vi "Derivative (DVR).vi"(4 "Type":enum16{"dy/dx vs x", "dx/dy vs y"}(ring), 7 "Data Value Reference in":refnum<data-value>, 8 "error in (no error)":errorcluster, 11 "dX in":refnum<data-value>) -> (0 "error out":errorcluster, 3 "dX out":refnum<data-value>)   [LabVIEW 2016, in "Retrieve and Visualize.lvclass"]
uses:
  Retrieve and Visualize.lvclass
  <userlib>/LevyLab/XY Utilities/subVIs/Derivative (multiple).vi
  <userlib>/LevyLab/XY Utilities/xy_utilities.lvlib
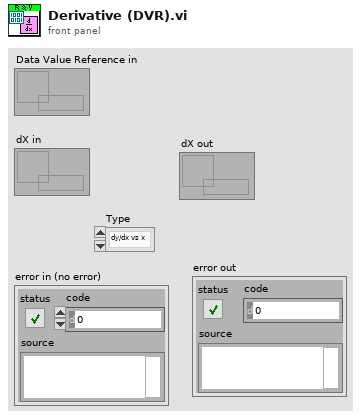
[diagram p1: front panel]
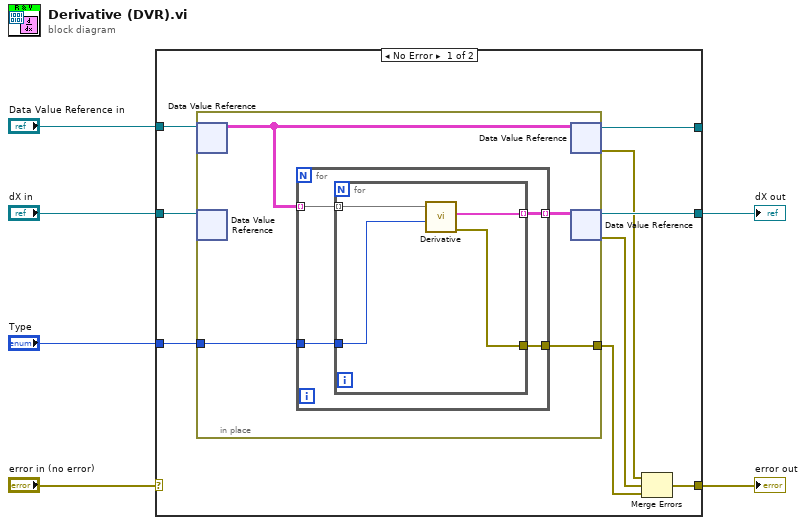
[diagram p0: block diagram]
diagram:
  n1 = case shown="No Error" "error in (no error)" {
    selector: "error in (no error)" -> [_ w28]
    tunnel: [w15 w29] -> _
    tunnel: "Data Value Reference in" -> [w14 w29]
    tunnel: "dX in" -> [w13 w30]
    tunnel: [w12 w30] -> w4
    tunnel: "Type" -> [w11 _]
    tunnel: [w8 w28] -> w1
    frame No Error {
      n2 = in-place {
        in-place-border: w11 -> [w18]
        in-place-border: [w17] -> w7
        n3 = in-place-dvr #1(w14) -> (w16:cluster{dbl[], dbl[]}[][][])  [unwired: 1 out]
        n4 = in-place-dvr #2(w13) -> ()  [unwired: 2 out]
        n5 = for {
          tunnel: [w23] -> w19 mode=indexing
          tunnel: w16 -> [w22] mode=indexing
          tunnel: w18 -> [w21]
          tunnel: [w20] -> w17
          n6 = for {
            tunnel: w22 -> [w26] mode=indexing
            tunnel: [w27] -> w23 mode=indexing
            tunnel: w21 -> [w25]
            tunnel: [w24] -> w20
            n7 = call-poly <userlib>:"Derivative.vi"("Type"=w25, "XY-data"=w26) -> ("error out"=w24:errorcluster, "Differential out"=w27:cluster{"X-array":dbl[], "Y-array":dbl[]}[])  [unwired: 7 in, 1 out]
          }
        }
        n8 = in-place-dvr #1(w16) -> (w15:refnum<data-value>, w10:errorcluster)
        n9 = in-place-dvr #2(w19) -> (w12:refnum<data-value>, w9:errorcluster)
      }
      n10 = Merge Errors(w10, w9, w7) -> (w8:errorcluster)
    }
    frame Error {
    }
  }
  "dX out" <- w4
  "error out" <- w1
